vi "launch tcp vi handler.vi"(8 "error in":errorcluster, 9 "command line arguments":T1, 10 "base path":path, 11 "labview directory":path) -> (0 "error out":errorcluster)   [LabVIEW 2013]
uses:
  arguments.ctl
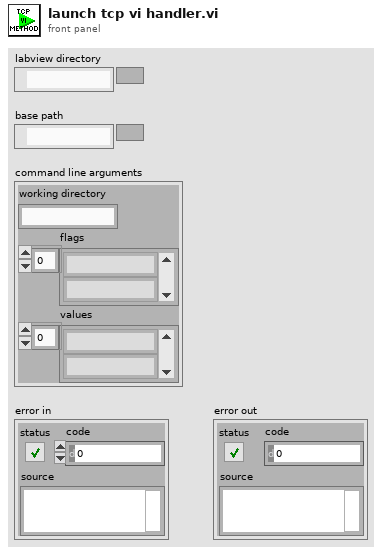
[diagram p1: front panel]
types:
  T1 = typedef "arguments.ctl" = cluster{"working directory":string, "flags":string[], "values":string[]}
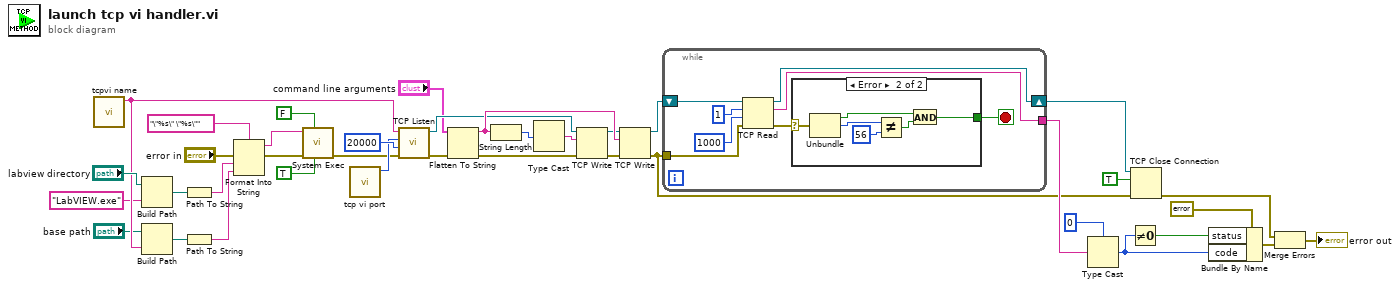
[diagram p0: block diagram]
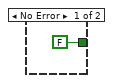
[diagram p2: hidden frame]
diagram:
  n1 = call "tcpvi name.vi"() -> ("tcpvi name"=w36:string)  [unwired: 11 in]
  n2 = Build Path(base path="labview directory", name or relative path="LabVIEW.exe" ("format string")) -> (appended path=w7:path)
  n3 = Build Path(base path="base path", name or relative path=w36) -> (appended path=w9:path)
  n4 = Path To String(path=w7) -> (string=w10:string)
  n5 = Path To String(path=w9) -> (string=w11:string)
  n6 = Format Into String(format string="\"%s\" \"%s\"", error in="error in", w10, w11) -> (resulting string=w14:string, error out=w13:errorcluster)  [unwired: 1 in]
  n7 = call <vilib>:"System Exec.vi"("run minimized? (F)"=TRUE, "wait until completion? (T)"=FALSE, "error in (no error)"=w13, "command line"=w14) -> ("error out"=w17:errorcluster)  [unwired: 4 in, 3 out]
  n8 = call "tcp vi port.vi"() -> ("port"=w18:u16)  [unwired: 11 in]
  n9 = call <vilib>:"TCP Listen.vi"("error in (no error)"=w17, "timeout ms (wait forever: -1)"=20000, "port"=w18, "service name"=w36) -> ("error out"=w20:errorcluster, "connection ID"=w28:refnum<k5>)  [unwired: 3 in, 3 out]
  n10 = Flatten To String(anything="command line arguments", error in (no error)=w20) -> (data string=w30:string, error out=w21:errorcluster)  [unwired: 2 in, 1 out]
  n11 = String Length(string=w30) -> (length=w31:i32)
  n12 = Type Cast(x=w31) -> (*(type *) &x=w32:string)  [unwired: 1 in]
  n13 = TCP Write(connection ID=w28, data in=w32, error in (no error)=w21) -> (connection ID out=w29:refnum<k5>, error out=w27:errorcluster)  [unwired: 1 in, 1 out]
  n14 = TCP Write(connection ID=w29, data in=w30, error in (no error)=w27) -> (connection ID out=w23:refnum<k5>, error out=w25:errorcluster)  [unwired: 1 in, 1 out]
  n15 = while {
    tunnel: w25 -> [w45]
    shift-right: [w44] -> w24
    shift-left: w23 -> [w46]
    tunnel: [w41] -> w33
    stop <- w39 stop-if-true
    n16 = TCP Read(connection ID=w46, bytes to read=1, error in (no error)=w45, 9:1000 ("timeout ms (25000)")) -> (connection ID out=w44:refnum<k5>, data out=w41:string, error out=w40:errorcluster)  [unwired: 1 in]
    n17 = case shown="Error" w40 {
      selector: w40 -> [_ w53]
      tunnel: [FALSE w48] -> w39
      frame No Error {
      }
      frame Error {
        n18 = Unbundle(w53) -> ("status"=w49:bool, "code"=w52:i32)  [unwired: 1 out]
        n19 = Not Equal?(x=w52, y=56) -> (x != y?=w50:bool)
        n20 = And(x=w49, y=w50) -> (x .and. y?=w48:bool)
      }
    }
  }
  n21 = Type Cast(type=i8 0, x=w33) -> (*(type *) &x=w3:i8)
  n22 = Not Equal To 0?(x=w3) -> (x != 0?=w2:bool)
  n23 = TCP Close Connection(connection ID=w24, abort (F)=TRUE, error in (no error)=w25) -> (error out=w35:errorcluster)  [unwired: 1 out]
  n24 = Bundle By Name(cluster=errorcluster {"status"=FALSE, "code"=0, "source"=""} ("error in"), "status"=w2, "code"=w3) -> (w1:errorcluster)
  n25 = Merge Errors(w35, w1) -> (→"error out":errorcluster)
